vi "ReadLogFile.vi"() -> ()   [LabVIEW 2009]
uses:
  LogData.ctl
panel:
  in  "Reset Search":bool
  in  "found in record":i32
  in  "Search":bool
  in  "stop 2":bool
  in  "Command Code":string
  out "Array":T1[](array[typedef])
  out "Record":i32
  in  "stop":bool
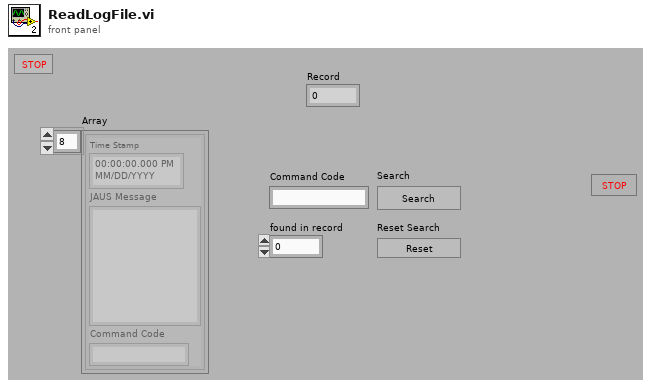
[diagram p1: front panel]
types:
  T1 = typedef "LogData.ctl" = cluster{"Time Stamp":timestamp, "JAUS Message":string, "Command Code":string}
  T2 = enum16{"open", "replace", "create", "open or create", "replace or create", "replace or create with confirmation"}
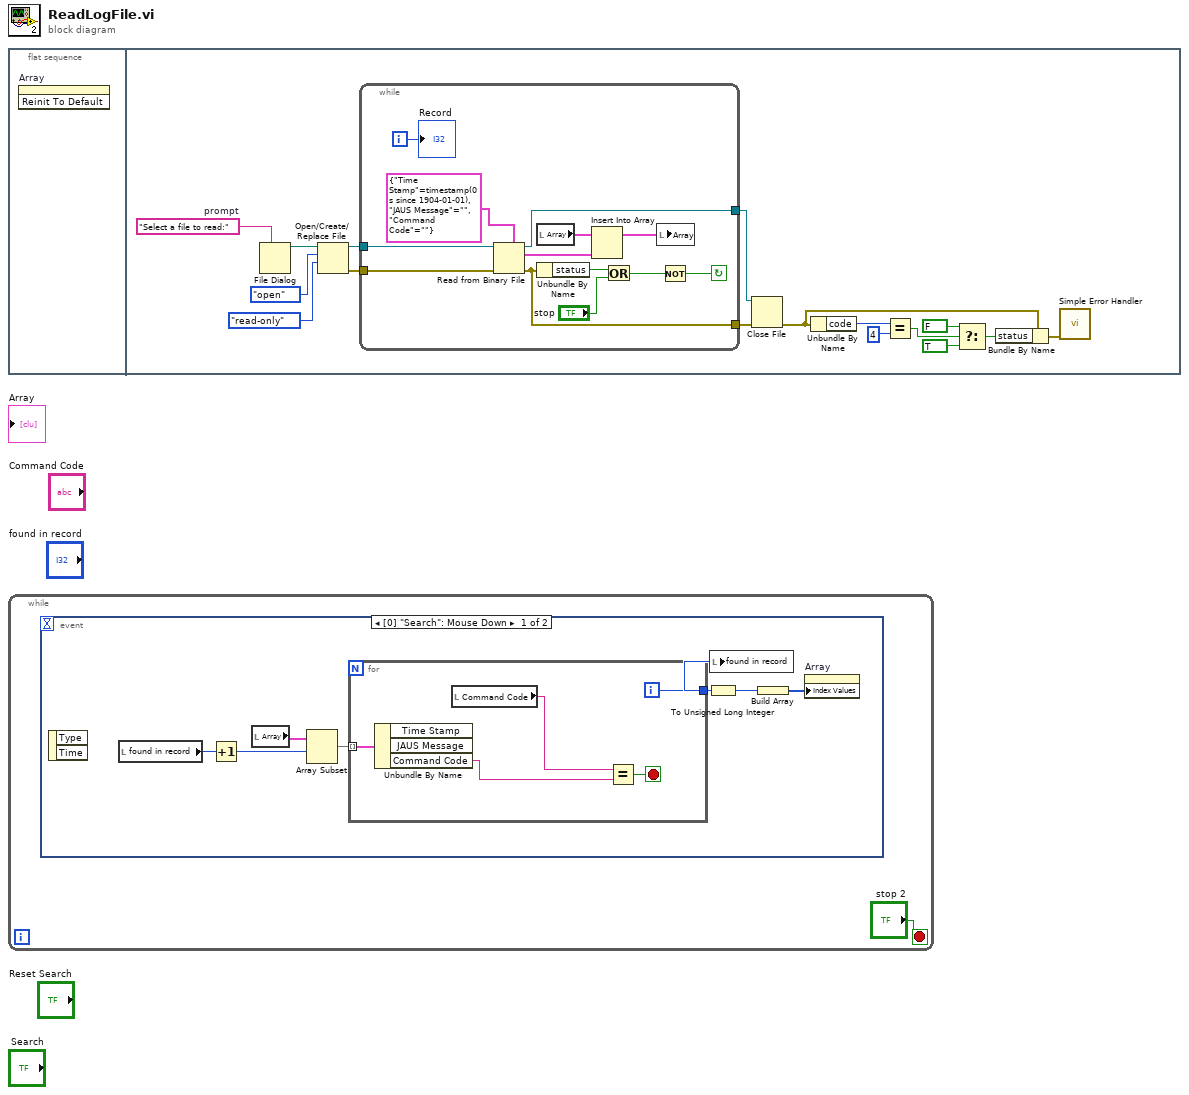
[diagram p0: block diagram]
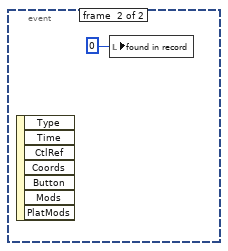
[diagram p2: hidden frame]
diagram:
  n1 = flat-sequence {
    frame #0 {
      n2 = invoke on="Array" class="Arr (strict)" method="Reinit To Default"() -> ()  [unwired: 3 in, 3 out]
    }
    frame #1 {
      w16 = "Select a file to read:"  # prompt
      n3 = File Dialog(7:w16) -> (3:w15:path)  [unwired: 1 in, 8 out]
      n4 = Open/Create/Replace File(file path (use dialog)=w15, operation (0:open)=T2."open", access (0:read/write)=enum16{"read/write", "read-only", "write-only"}."read-only") -> (refnum out=w12:refnum<file>, error out=w11:errorcluster)  [unwired: 1 in, 3 out]
      n5 = while {
        tunnel: w12 -> [w22]
        tunnel: w11 -> [w19]
        tunnel: [w20] -> w2
        tunnel: [w21] -> w1
        i -> [w23]
        stop <- w25 continue-if-true
        n6 = Read from Binary File(5:T1 {"Time Stamp"=timestamp(0 s since 1904-01-01), "JAUS Message"="", "Command Code"=""} ("LogData"), 8:w19, 11:w22) -> (0:w20:errorcluster, 2:w17:T1, 3:w21:refnum<file>)  [unwired: 3 in, 1 out]
        n7 = local read "Array"() -> (w29:T1[])
        n8 = Unbundle By Name(w20) -> ("status"=w26:bool)
        n9 = Insert Into Array(array=w29, new element=w17) -> (w24:T1[])  [unwired: 1 in]
        n10 = Or(x=w26, y="stop") -> (x .or. y?=w27:bool)
        n11 = local write "Array"(w24) -> ()
        n12 = Not(x=w27) -> (.not. x?=w25:bool)
        "Record" <- w23
      }
      n13 = Close File(refnum=w1, error in=w2) -> (error out=w5:errorcluster)  [unwired: 1 out]
      n14 = Unbundle By Name(w5) -> ("code"=w10:i32)
      n15 = Equal?(x=w10, y=4) -> (x = y?=w8:bool)
      n16 = Select(t=FALSE, s=w8, f=TRUE) -> (s? t:f=w4:bool)
      n17 = Bundle By Name(cluster=w5, "status"=w4) -> (w3:errorcluster)
      n18 = call <vilib>:"Simple Error Handler.vi"("error in (no error)"=w3) -> ()  [unwired: 4 in, 5 out]
    }
  }
  n19 = while {
    stop <- "stop 2" stop-if-true
    n20 = event shown="[0] \"Search\": Mouse Down" {
      selector: _ -> [_ _]
      dyn-events: _ -> [_ _]
      timeout: _ -> [_ _]
      event #0 {
        n21 = event-data() -> ()  [unwired: 1 in, 2 out]
        n22 = local read "found in record"() -> (w35:i32)
        n23 = Increment(x=w35) -> (x+1=w31:i32)
        n24 = local read "Array"() -> (w36:T1[])
        n25 = Array Subset(array=w36, index=w31) -> (w37:T1[])  [unwired: 1 in]
        n26 = for {
          tunnel: w37 -> [w42] mode=indexing
          tunnel: [w40] -> w33
          i -> [w40]
          stop <- w41 stop-if-true
          n27 = Unbundle By Name(w42) -> ("Command Code"=w38:string)  [unwired: 2 out]
          n28 = local read "Command Code"() -> (w39:string)
          n29 = Equal?(x=w39, y=w38) -> (x = y?=w41:bool)
        }
        n30 = To Unsigned Long Integer(number=w33) -> (unsigned 32bit integer=w32:u32)
        n31 = local write "found in record"(w33) -> ()
        n32 = Build Array(w32) -> (w34:u32[])
        n33 = property on="Array" class="Arr (strict)"("Index Values"=w34) -> ()  [unwired: 2 in, 2 out]
      }
      event #1 {
        n34 = event-data() -> ()  [unwired: 1 in, 7 out]
        n35 = local write "found in record"(0 ("found in record")) -> ()
      }
    }
  }
